vi "Compressor.vi"   [LabVIEW 2014]
uses:
  Begin/Global RefNums.vi
  <vilib>/Rock Robotics/WPI/Compressor/WPI_CompressorGetSetRefNum.vi
types:
  T1 = typedef "WPI_CompressorDevRef.ctl" = cluster{"DevStatus":errorcluster, "Pneumatics Control Module":u8}
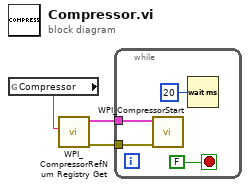
[diagram p0: block diagram]
diagram:
  n1 = global read "Global RefNums.vi" "Compressor"() -> (w3:string)
  n2 = call <vilib>:"WPI_CompressorRefNum Registry Get.vi"("refnum name"=w3) -> ("error out"=w1:errorcluster, "CompressorDevRef"=w2:T1)  [unwired: 9 in]
  n3 = while {
    tunnel: w2 -> [w5]
    tunnel: w1 -> [w4]
    stop <- FALSE stop-if-true
    n4 = call <vilib>:"WPI_CompressorStart.vi"("error in (no error)"=w4, "CompressorDevRef"=w5) -> ()  [unwired: 8 in, 2 out]
    n5 = Wait (ms)(milliseconds to wait=u32 20) -> ()  [unwired: 1 out]
  }
